vi "User_manager.vi"() -> ()   [LabVIEW 2020]
uses:
  Global1.vi
  <vilib>/addons/database/Connection.llb/DB Tools Open Connec (String).vi
  <vilib>/addons/database/Connection.llb/Conn Execute.vi
  <vilib>/addons/database/Recordset.llb/Rec Fetch Recordset Data (R).vi
  <vilib>/addons/database/NI_Database_API.lvlib
panel:
  out "用户信息":string[][](table)
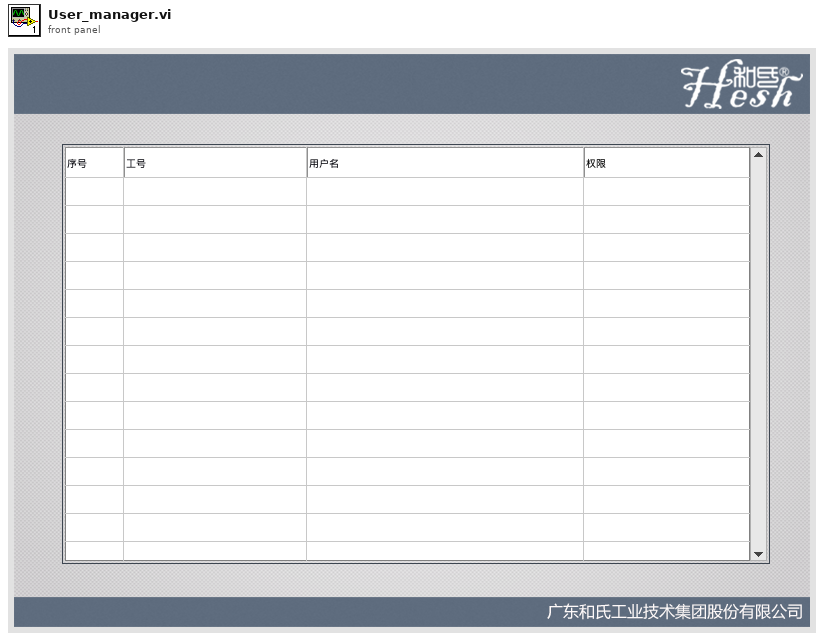
[diagram p1: front panel]
types:
  T1 = enum32{"Invalid", "Standard", "Closed", "Hidden", "Minimized", "Maximized"}
  T2 = typedef "NI_Database_API.lvlib/Conn ObjectReference.ctl" = refnum<k1>
  T3 = typedef "NI_Database_API.lvlib/Rec ObjectReference.ctl" = refnum<k1>
  T4 = typedef "LVPoint32TypeDef.ctl" = cluster{"Horizontal":i32, "Vertical":i32}
  T5 = typedef "LVRowAndColumnTypeDef.ctl" = cluster{"Row":i32, "Column":i32}
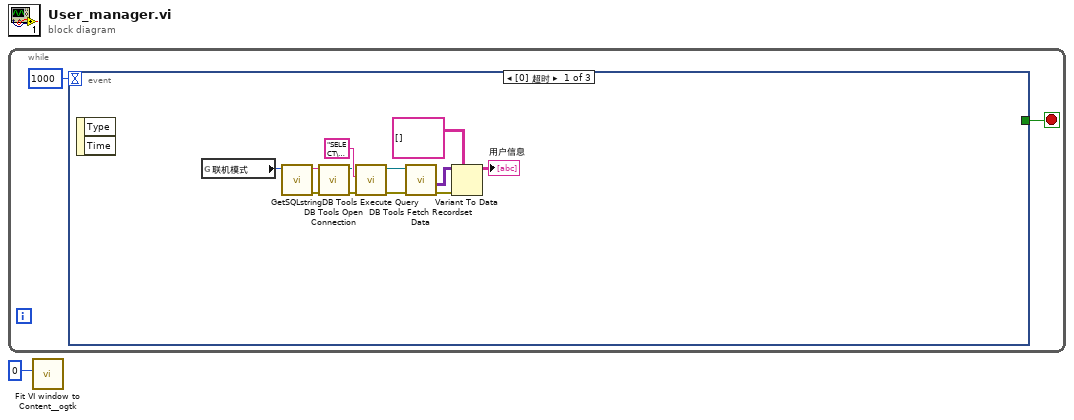
[diagram p0: block diagram]
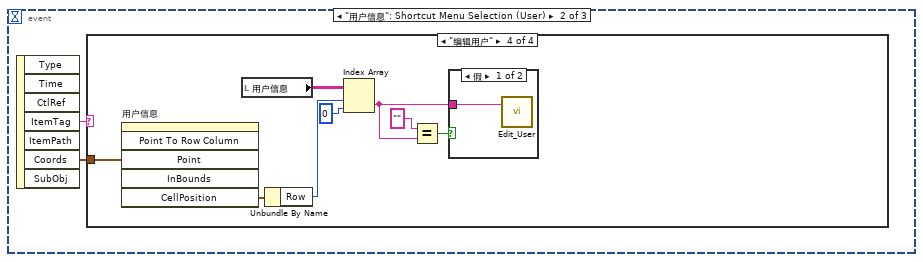
[diagram p2: hidden frame]
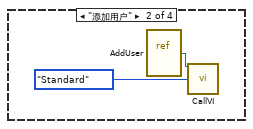
[diagram p4: hidden frame]
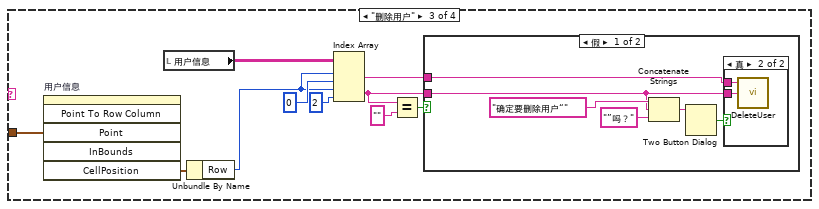
[diagram p5: hidden frame]
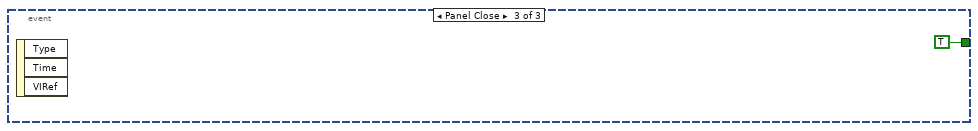
[diagram p9: hidden frame]
diagram:
  n1 = while {
    stop <- w2 stop-if-true
    n2 = event shown="[0] 超时" {
      selector: _ -> [_ _ _]
      dyn-events: _ -> [_ _ _]
      timeout: 1000 -> [_ _ _]
      tunnel: [_ _ TRUE] -> w2
      event Timeout {
        n3 = event-data() -> ()  [unwired: 1 in, 2 out]
        n4 = global read "Global1.vi" "联机模式"() -> (w6:enum16{"单机", "联网"})
        n5 = call "GetSQLstring.vi"("联机模式"=w6) -> ("错误输出"=w5:errorcluster, "连接字符串"=w7:string)  [unwired: 9 in]
        n6 = call-poly <vilib>:"DB Tools Open Connection.vi"("error in (no error)"=w5, "connection information"=w7) -> ("error out"=w4:errorcluster, "connection reference"=w8:T2)  [unwired: 6 in]
        n7 = call-poly <vilib>:"DB Tools Execute Query.vi"("error in (no error)"=w4, "SQL query"="SELECT\ndbo.[User].USER_ID,\ndbo.[User].USER_EMPLOYEE_ID,\ndbo.[User].USER_NAME,\ndbo.[User].USER_PERMIT\n\nFROM\ndbo.[User]", "connection reference"=w8) -> ("error out"=w13:errorcluster, "recordset reference"=w12:T3)  [unwired: 5 in]
        n8 = call-poly <vilib>:"DB Tools Fetch Recordset Data.vi"("error in (no error)"=w13, "recordset reference"=w12) -> ("error out"=w11:errorcluster, "recordset data"=w10:variant[][])  [unwired: 3 in, 1 out]
        n9 = Variant To Data(error in=w11, type=string[][] [], Variant=w10) -> (data=→"用户信息":string[][])  [unwired: 1 out]
      }
      event "用户信息": Shortcut Menu Selection (User) {
        n10 = event-data() -> ("ItemTag"=w17:string, "Coords"=w16:T4)  [unwired: 1 in, 5 out]
        n11 = case shown="\"编辑用户\"" w17 {
          tunnel: w16 -> [_ _ w29 w41]
          frame Default {
          }
          frame "添加用户" {
            n12 = vi-ref "AddUser.vi"() -> (w19:refnum<vi>)
            n13 = call "CallVI.vi"("VI引用"=w19, "状态"=T1."Standard") -> ()  [unwired: 11 in, 3 out]
          }
          frame "删除用户" {
            n14 = invoke on="用户信息" class="Tbl (严格)" method="Point To Row Column"("Point"=w29) -> ("CellPosition"=w28:T5)  [unwired: 5 in, 5 out]
            n15 = local read "用户信息"() -> (w27:string[][])
            n16 = Unbundle By Name(w28) -> ("Row"=w25:i32)
            n17 = Index Array(array=w27, index (row) #1=w25, index (col) #1=0 ("禁用的索引 (列)"), index (row) #2=w25, index (col) #2=2 ("禁用的索引 (列)")) -> (element #1=w23:string, element #2=w22:string)
            n18 = Equal?(x=w22, y="" ("元素")) -> (x = y?=w20:bool)
            n19 = case shown="假" w20 {
              tunnel: w22 -> [w31 _]
              tunnel: w23 -> [w30 _]
              frame False {
                n20 = Concatenate Strings("确定要删除用户“" ("字符串"), w31, "”吗？" ("字符串")) -> (w33:string)
                n21 = Two Button Dialog(message=w33) -> (T button?=w32:bool)  [unwired: 2 in]
                n22 = case shown="真" w32 {
                  tunnel: w31 -> [_ w37]
                  tunnel: w30 -> [_ w36]
                  frame False {
                  }
                  frame True {
                    n23 = call "DeleteUser.vi"("User_Name"=w37, "ID"=w36) -> ()  [unwired: 3 in, 1 out]
                  }
                }
              }
              frame True {
              }
            }
          }
          frame "编辑用户" {
            n24 = invoke on="用户信息" class="Tbl (严格)" method="Point To Row Column"("Point"=w41) -> ("CellPosition"=w45:T5)  [unwired: 5 in, 5 out]
            n25 = local read "用户信息"() -> (w44:string[][])
            n26 = Unbundle By Name(w45) -> ("Row"=w43:i32)
            n27 = Index Array(array=w44, index (row)=w43, index (col)=0 ("禁用的索引 (列)")) -> (element=w38:string)
            n28 = Equal?(x="" ("元素"), y=w38) -> (x = y?=w40:bool)
            n29 = case shown="假" w40 {
              tunnel: w38 -> [w46 _]
              frame False {
                n30 = call "Edit_User.vi"("用户ID"=w46) -> ()  [unwired: 2 in]
              }
              frame True {
              }
            }
          }
        }
      }
      event Panel Close {
        n31 = event-data() -> ()  [unwired: 1 in, 3 out]
      }
    }
  }
  n32 = call <userlib>:"Fit VI window to Content__ogtk.vi"("border spacing (2 px)"=0) -> ()  [unwired: 5 in, 2 out]
